vi "Config Arm Event.vi"(6 "Arm Input Event":string="0", 8 "error in":errorcluster, 9 "Channel (Channel A)":T1, 10 "Node In":string, 11 "VISA resource name":refnum<visa-resource-name>) -> (0 "error out":errorcluster, 2 "Node Out":string, 3 "VISA resource name out":refnum<visa-resource-name>, 4 "Command String":string)   [LabVIEW 2012, in "Keithley 2600 Series.lvlib"]
doc: "This VI configures the arm event of the SMU in the advanced trigger model.\n\n<b>Functions and Attributes Used</b>\nsmuX.trigger.arm.stimulus"
uses:
  Keithley 2600 Series.lvlib
  Private/GlobalVariables.vi
  Channel.ctl
panel:
  # "(c) 2008 Keithley Instruments, Inc.  ALL RIGHTS RESERVED."
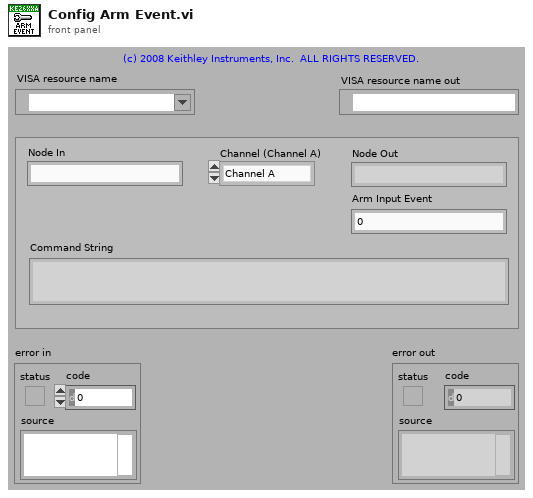
[diagram p1: front panel]
types:
  T1 = typedef "Keithley 2600 Series.lvlib/Channel.ctl" = enum32{"Channel A", "Channel B"}
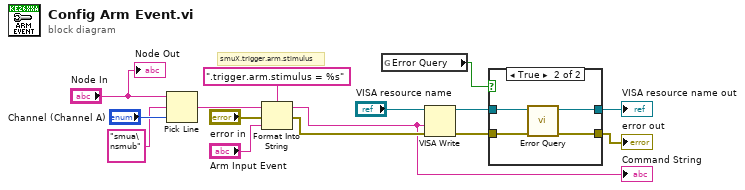
[diagram p0: block diagram]
diagram:
  # "smuX.trigger.arm.stimulus"
  n1 = Pick Line(string ("")="Node In", multi-line string="smua\nsmub", line index="Channel (Channel A)") -> (output string=w11:string)
  n2 = Format Into String(format string=".trigger.arm.stimulus = %s", initial string=w11, error in="error in", "Arm Input Event") -> (resulting string=w1:string, error out=w8:errorcluster)
  "Command String" <- w1
  n3 = global read "GlobalVariables.vi" "Error Query"() -> (w6:bool)
  n4 = VISA Write(VISA resource name="VISA resource name", write buffer=w1, error in (no error)=w8) -> (VISA resource name out=w5:refnum<visa-resource-name>, error out=w4:errorcluster)  [unwired: 1 out]
  n5 = case shown="True" w6 {
    tunnel: w5 -> [w17 w21]
    tunnel: w4 -> [w16 w20]
    tunnel: [w17 w19] -> w3
    tunnel: [w16 w18] -> w2
    frame False {
    }
    frame True {
      n6 = call "Error Query.vi"("error in (no error)"=w20, "VISA resource name"=w21) -> ("error out"=w18:errorcluster, "VISA resource name out"=w19:refnum<visa-resource-name>)  [unwired: 8 out]
    }
  }
  "VISA resource name out" <- w3
  "error out" <- w2
  "Node Out" <- "Node In"
